vi "Parse Token.vi"(10 "Token":T1, 11 "Line":string) -> (2 "Value":string, 3 "Name":string)   [LabVIEW 2017, in "LabVIEW-Config.lvlib" / "LabVIEW-Config.lvclass"]
uses:
  LabVIEW-Config.lvclass
  LineToken.ctl
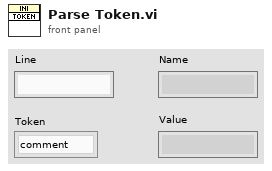
[diagram p1: front panel]
types:
  T1 = typedef "LabVIEW-Config.lvlib/LabVIEW-Config.lvclass/LineToken.ctl" = enum8{"comment", "section", "key", "more"}
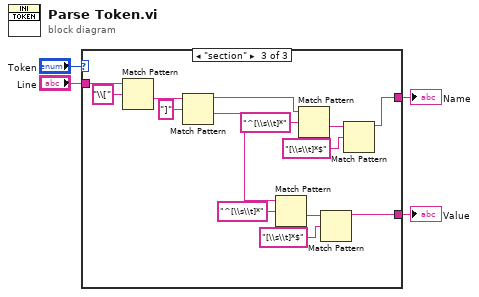
[diagram p0: block diagram]
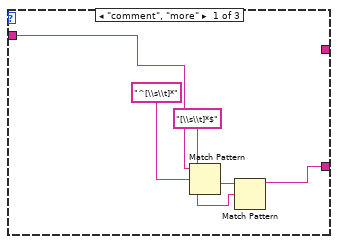
[diagram p2: hidden frame]
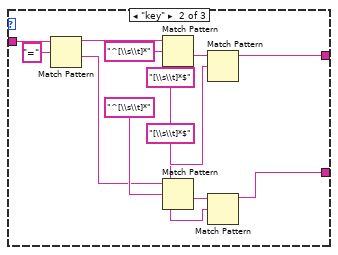
[diagram p3: hidden frame]
diagram:
  n1 = case shown="\"section\"" "Token" {
    tunnel: "Line" -> [w6 w16 w32]
    tunnel: [_ w15 w22] -> w2
    tunnel: [w5 w10 w27] -> w1
    frame "comment", "more" {
      n2 = Match Pattern(string=w6, regular expression="^[\\s\\t]*") -> (after substring=w9:string)  [unwired: 1 in, 3 out]
      n3 = Match Pattern(string=w9, regular expression="[\\s\\t]*$") -> (before substring=w5:string)  [unwired: 1 in, 3 out]
    }
    frame "key" {
      n4 = Match Pattern(string=w16, regular expression="=") -> (before substring=w17:string, after substring=w11:string)  [unwired: 1 in, 2 out]
      n5 = Match Pattern(string=w17, regular expression="^[\\s\\t]*") -> (after substring=w20:string)  [unwired: 1 in, 3 out]
      n6 = Match Pattern(string=w11, regular expression="^[\\s\\t]*") -> (after substring=w12:string)  [unwired: 1 in, 3 out]
      n7 = Match Pattern(string=w20, regular expression="[\\s\\t]*$") -> (before substring=w15:string)  [unwired: 1 in, 3 out]
      n8 = Match Pattern(string=w12, regular expression="[\\s\\t]*$") -> (before substring=w10:string)  [unwired: 1 in, 3 out]
    }
    frame "section" {
      n9 = Match Pattern(string=w32, regular expression="\\[") -> (after substring=w33:string)  [unwired: 1 in, 3 out]
      n10 = Match Pattern(string=w33, regular expression="]") -> (before substring=w23:string, after substring=w28:string)  [unwired: 1 in, 2 out]
      n11 = Match Pattern(string=w28, regular expression="^[\\s\\t]*") -> (after substring=w29:string)  [unwired: 1 in, 3 out]
      n12 = Match Pattern(string=w23, regular expression="^[\\s\\t]*") -> (after substring=w26:string)  [unwired: 1 in, 3 out]
      n13 = Match Pattern(string=w29, regular expression="[\\s\\t]*$") -> (before substring=w27:string)  [unwired: 1 in, 3 out]
      n14 = Match Pattern(string=w26, regular expression="[\\s\\t]*$") -> (before substring=w22:string)  [unwired: 1 in, 3 out]
    }
  }
  "Value" <- w1
  "Name" <- w2
